vi "Write Value.vi"(8 "error in (no error)":errorcluster, 10 "Value":i32, 11 "int32 in":refnum<class "sint32.lvclass">) -> (0 "error out":errorcluster, 3 "int32 out":refnum<class "sint32.lvclass">)   [LabVIEW 2020, in "Protobuf RAW.lvlib" / "sint32.lvclass"]
uses:
  sint32.lvclass
  sint32.lvclass/sint32.ctl
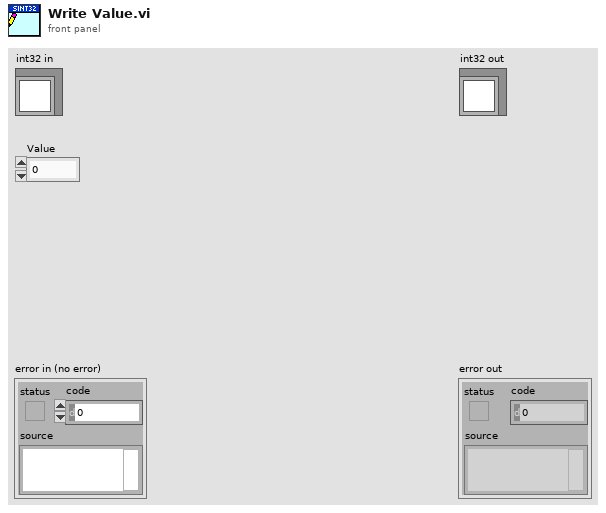
[diagram p1: front panel]
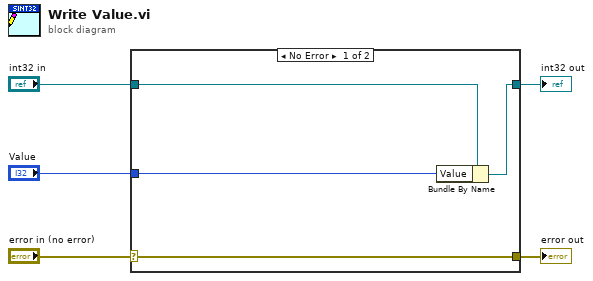
[diagram p0: block diagram]
diagram:
  n1 = case shown="No Error" "error in (no error)" {
    selector: "error in (no error)" -> [w9 w10]
    tunnel: [w9 w10] -> w4
    tunnel: [w7 w11] -> w2
    tunnel: "int32 in" -> [w8 w11]
    tunnel: "Value" -> [w6 _]
    frame No Error {
      n2 = Bundle By Name(cluster=w8, "Value"=w6) -> (w7:refnum<class "sint32.lvclass">)
    }
    frame Error {
    }
  }
  "error out" <- w4
  "int32 out" <- w2
